vi "SW_Gen_2D_Histogram_2.vi"(6 "Pic. ref. for sizing":refnum<vi>, 7 "Pixels per mm":dbl=3.2, 8 "error in (no error)":errorcluster, 9 "Y coord array":dbl[](array[numeric]), 10 "X coord array":dbl[](array[numeric]), 11 "Bounds, pix":T6={"Width"=320, "Height"=320}) -> (0 "B/W picture (density)":picture, 1 "24-bit b/w density pixmap":u32[][](array[numeric]), 2 "Colored picture":picture, 3 "24-bit color pixmap":u32[][](array[numeric]))   [LabVIEW 2018, in "Tracker.lvlib"]
uses:
  Tracker.lvlib
  <vilib>/Utility/miscctls.llb/LVBoundsTypeDef.ctl
  <vilib>/Heliosphere Research LLC/Advanced Plotting Toolkit/api_plotting/Histogram2DProperties.ctl
  <vilib>/Heliosphere Research LLC/Advanced Plotting Toolkit/properties/Colormap.ctl
  <vilib>/Heliosphere Research LLC/Advanced Plotting Toolkit/properties/Colormap_Map.ctl
  <vilib>/Heliosphere Research LLC/Advanced Plotting Toolkit/properties/Colormap_Scaling.ctl
  <vilib>/Heliosphere Research LLC/Advanced Plotting Toolkit/properties/Display.ctl
  <vilib>/Heliosphere Research LLC/Advanced Plotting Toolkit/api_core/NewPlotType.ctl
  <vilib>/Heliosphere Research LLC/Advanced Plotting Toolkit/api_plotting/Histogram2DRange.ctl
  <vilib>/Heliosphere Research LLC/Advanced Plotting Toolkit/api_core/NewPlotProperties.ctl
  <vilib>/Heliosphere Research LLC/Advanced Plotting Toolkit/typedefs/PlotColor.ctl
  <vilib>/Heliosphere Research LLC/Advanced Plotting Toolkit/api_core/NewPlotScales.ctl
  <vilib>/Heliosphere Research LLC/Advanced Plotting Toolkit/api_plotting/Histogram2D_Automatic.vi
  <vilib>/Heliosphere Research LLC/Advanced Plotting Toolkit/Advanced Plotting Toolkit.lvlib
panel:
  in  "Histogram (colored) props":T1={"Normalize"=FALSE, "Colormap"={"Map"=enum."Rainbow", "Value Min"=nan, "Value Max"=nan, "Scaling"=enum."Default", "Reverse"=FALSE}, "Display"={"Alpha"=1.0, "Z Order"=nan}}
  in  "Histogram (B/W) props":T1={"Normalize"=FALSE, "Colormap"={"Map"=enum."White-Black", "Value Min"=nan, "Value Max"=nan, "Scaling"=enum."Default", "Reverse"=TRUE}, "Display"={"Alpha"=nan, "Z Order"=nan}}
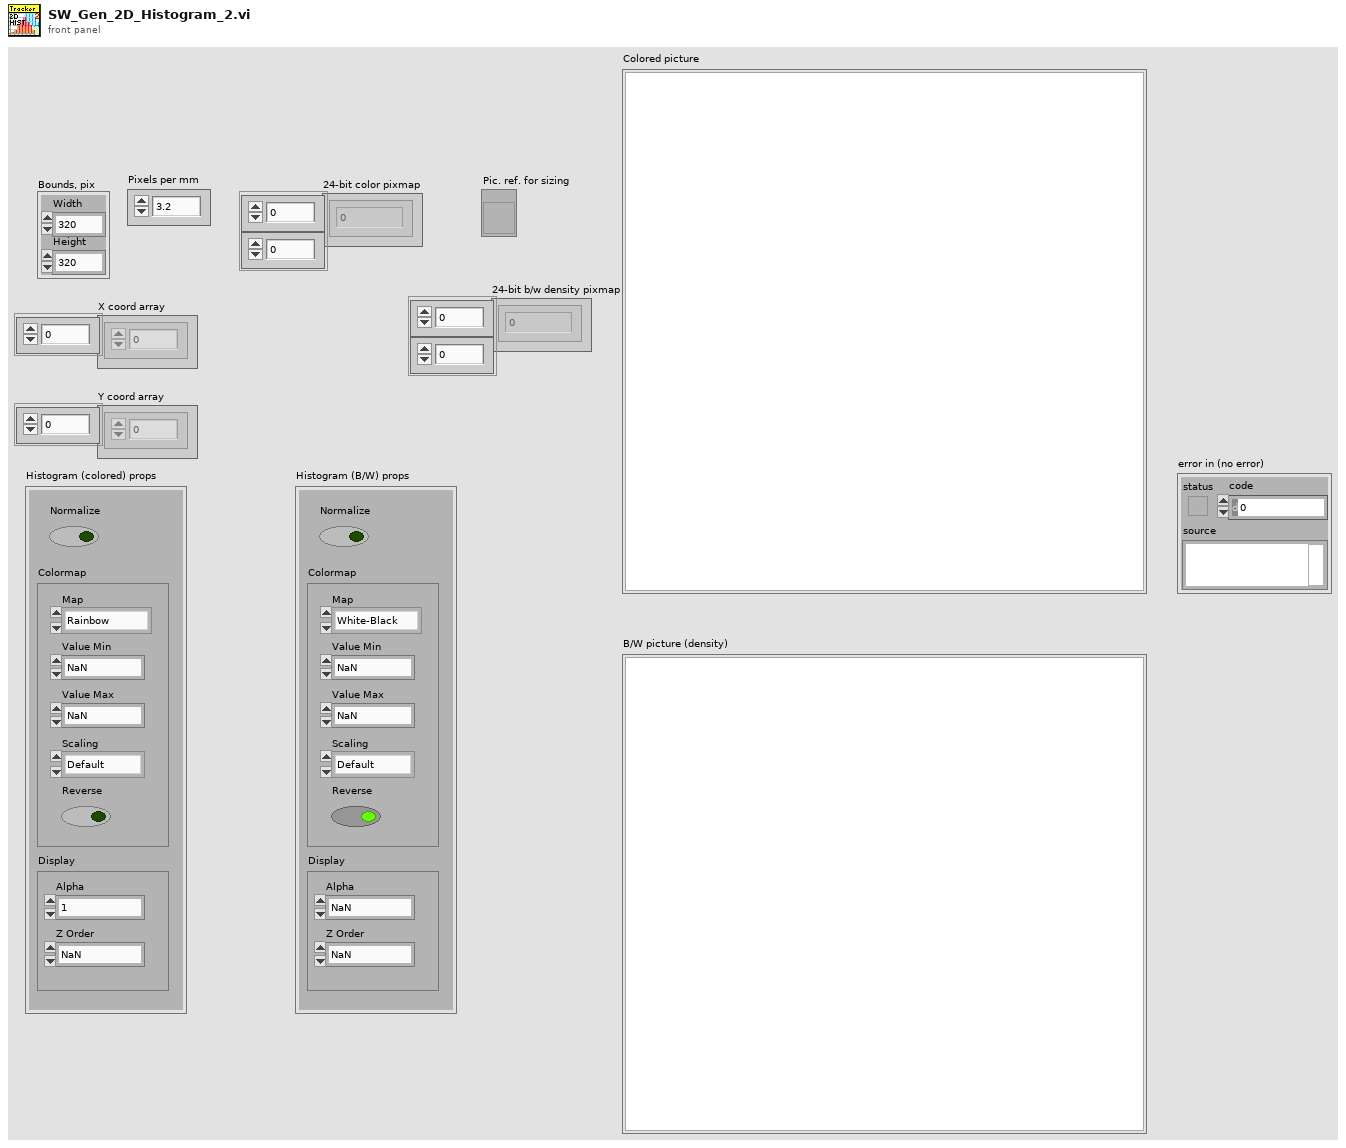
[diagram p1: front panel]
types:
  T1 = typedef "Advanced Plotting Toolkit.lvlib/Histogram2DProperties.ctl" = cluster{"Normalize":bool, "Colormap":T2, "Display":T5}
  T2 = typedef "Advanced Plotting Toolkit.lvlib/Colormap.ctl" = cluster{"Map":T3, "Value Min":dbl, "Value Max":dbl, "Scaling":T4, "Reverse":bool}
  T3 = typedef "Advanced Plotting Toolkit.lvlib/Colormap_Map.ctl" = enum16{"Automatic", "Rainbow", "Hot and Cold", "White-Black", "White-Blue", "White-Green", "White-Red", "Fire", "Water", "Earth", "Air", "Pastel", "Banded", "Stepped"}
  T4 = typedef "Advanced Plotting Toolkit.lvlib/Colormap_Scaling.ctl" = enum16{"Default"}
  T5 = typedef "Advanced Plotting Toolkit.lvlib/Display.ctl" = cluster{"Alpha":dbl, "Z Order":dbl}
  T6 = typedef "LVBoundsTypeDef.ctl" = cluster{"Width":u32, "Height":u32}
  T7 = typedef "Advanced Plotting Toolkit.lvlib/NewPlotScales.ctl" = enum16{"Default", "Linear", "Log", "Symlog"}
  T8 = typedef "Advanced Plotting Toolkit.lvlib/NewPlotProperties.ctl" = cluster{"Background Color":T9, "Axis Background":T9, "Left Margin":dbl, "Right Margin":dbl, "Bottom Margin":dbl, "Top Margin":dbl, "Aspect Ratio":dbl}
  T9 = typedef "Advanced Plotting Toolkit.lvlib/PlotColor.ctl" = u32
  T10 = typedef "Advanced Plotting Toolkit.lvlib/Histogram2DRange.ctl" = cluster{"X Min":dbl, "X Max":dbl, "Y Min":dbl, "Y Max":dbl}
  T11 = typedef "Advanced Plotting Toolkit.lvlib/NewPlotType.ctl" = enum16{"Rectangular Axes", "Polar Axes"}
  T12 = typedef "Advanced Plotting Toolkit.lvlib/PlotID.ctl" = i32
  T13 = typedef "imagedata.ctl" = cluster{"image type":i32, "image depth":i32, "image":u8[], "mask":u8[], "colors":u32[], "Rectangle":cluster{"left":i16, "top":i16, "right":i16, "bottom":i16}}
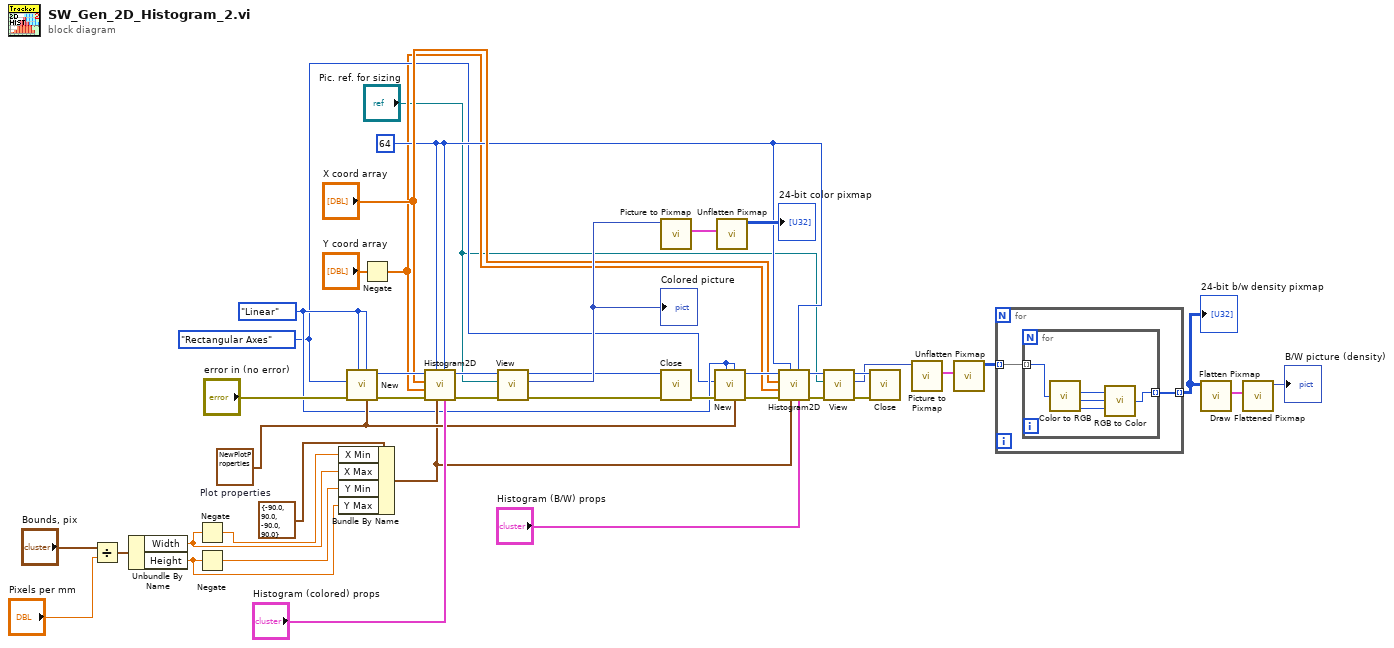
[diagram p0: block diagram]
diagram:
  w8 = NewPlotScales."Linear" ("X Axis Scale")
  w25 = T8 {"Background Color"=2147483647, "Axis Background"=2147483647, "Left Margin"=0.0, "Right Margin"=0.0, "Bottom Margin"=0.0, "Top Margin"=0.0, "Aspect Ratio"=1.0}  # Plot properties
  w6 = NewPlotType."Rectangular Axes" ("Plot Type")
  w7 = 64 ("Y Bins")
  n1 = Divide(x="Bounds, pix", y="Pixels per mm") -> (x/y=w38:cluster{"Width":dbl, "Height":dbl})
  n2 = Unbundle By Name(w38) -> ("Width"=w39:dbl, "Height"=w40:dbl)
  n3 = Negate(x=w39) -> (-x=w41:dbl)
  n4 = Negate(x=w40) -> (-x=w42:dbl)
  n5 = Bundle By Name(cluster=T10 {"X Min"=-90.0, "X Max"=90.0, "Y Min"=-90.0, "Y Max"=90.0} ("Data Range"), "X Min"=w41, "X Max"=w39, "Y Min"=w42, "Y Max"=w40) -> (w15:T10)
  n6 = call <vilib>:"New.vi"("Properties"=w25, "Y Axis Scale"=w8, "X Axis Scale"=w8, "error in (no error)"="error in (no error)", "Plot Type"=w6) -> ("error out"=w31:errorcluster, "Plot ID"=w29:T12)  [unwired: 5 in]
  n7 = Negate(x="Y coord array") -> (-x=w4:dbl[])
  n8 = call-poly <vilib>:"Histogram2D.vi"("Properties"="Histogram (colored) props", "Y Bins"=w7, "Data Range"=w15, "X Bins"=w7, "error in (no error)"=w31, "Y Data"=w4, "X Data"="X coord array", "Plot ID"=w29) -> ("error out"=w32:errorcluster, "Plot ID Out"=w3:T12)  [unwired: 2 in]
  n9 = call <vilib>:"View.vi"("error in (no error)"=w32, "Ref for Sizing"="Pic. ref. for sizing", "Plot ID"=w3) -> ("error out"=w34:errorcluster, "Picture"=w35:picture, "Plot ID Out"=w33:T12)  [unwired: 6 in]
  "Colored picture" <- w35
  n10 = call <vilib>:"Picture to Pixmap.vi"("picture"=w35) -> ("image data"=w36:T13)  [unwired: 9 in, 1 out]
  n11 = call <vilib>:"Close.vi"("error in (no error)"=w34, "Plot ID"=w33) -> ("error out"=w17:errorcluster)  [unwired: 9 in]
  n12 = call <vilib>:"New.vi"("Properties"=w25, "Y Axis Scale"=w8, "X Axis Scale"=w8, "error in (no error)"=w17, "Plot Type"=w6) -> ("error out"=w16:errorcluster, "Plot ID"=w24:T12)  [unwired: 5 in]
  n13 = call <vilib>:"Unflatten Pixmap.vi"("image data"=w36) -> ("24-bit pixmap"=→"24-bit color pixmap":u32[][])  [unwired: 4 in, 6 out]
  n14 = call-poly <vilib>:"Histogram2D.vi"("Properties"="Histogram (B/W) props", "Y Bins"=w7, "Data Range"=w15, "X Bins"=w7, "error in (no error)"=w16, "Y Data"=w4, "X Data"="X coord array", "Plot ID"=w24) -> ("error out"=w21:errorcluster, "Plot ID Out"=w20:T12)  [unwired: 2 in]
  n15 = call <vilib>:"View.vi"("error in (no error)"=w21, "Ref for Sizing"="Pic. ref. for sizing", "Plot ID"=w20) -> ("error out"=w19:errorcluster, "Picture"=w11:picture, "Plot ID Out"=w18:T12)  [unwired: 6 in]
  n16 = call <vilib>:"Close.vi"("error in (no error)"=w19, "Plot ID"=w18) -> ()  [unwired: 9 in, 1 out]
  n17 = call <vilib>:"Picture to Pixmap.vi"("picture"=w11) -> ("image data"=w14:T13)  [unwired: 9 in, 1 out]
  n18 = call <vilib>:"Unflatten Pixmap.vi"("image data"=w14) -> ("24-bit pixmap"=w13:u32[][])  [unwired: 4 in, 6 out]
  n19 = for {
    tunnel: w13 -> [w44] mode=indexing
    tunnel: [w43] -> w1 mode=indexing
    n20 = for {
      tunnel: w44 -> [w49] mode=indexing
      tunnel: [w46] -> w43 mode=indexing
      n21 = call <vilib>:"Color to RGB.vi"("Color"=w49) -> ("R"=w48:u8, "G"=w45:u8, "B"=w47:u8)  [unwired: 1 out]
      n22 = call <vilib>:"RGB to Color.vi"("B"=w47, "G"=w45, "R"=w48) -> ("Color"=w46:u32)
    }
  }
  "24-bit b/w density pixmap" <- w1
  n23 = call <vilib>:"Flatten Pixmap.vi"("24-bit pixmap"=w1) -> ("image data"=w12:T13)  [unwired: 10 in]
  n24 = call <vilib>:"Draw Flattened Pixmap.vi"("image data"=w12) -> ("new picture"=→"B/W picture (density)":picture)  [unwired: 8 in]
